vi "Bundler_Selected Element.vi"(7 "Action":T1(ring)=enum."Wire Properties", 11 "Affected Items":T2) -> (0 "Display String":string, 1 "Selected Element Name":string, 2 "index of element":i32, 3 "Selected Element Term Refnum":refnum<vi>, 4 "last element":bool, 6 "first element":bool)   [LabVIEW 2023]
uses:
  top/BundleMagic.ctl
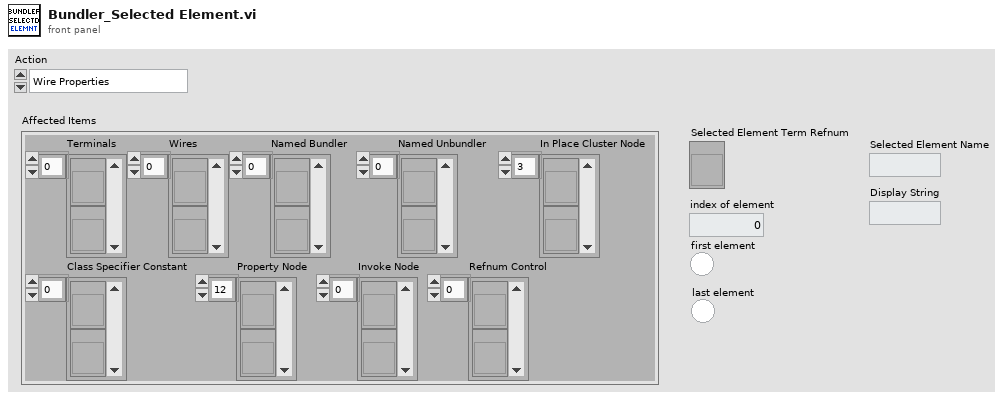
[diagram p1: front panel]
types:
  T1 = enum16{"[NONE]", "Wire Bundle", "Wire Unbundle", "Terminal Unbundle", "Terminal Bundle", "Bundler Move Up", "Bundler Move Down", "Bundler Insert", "Bundler Remove", "Bundler Remove Unwired", "Bundler Rearrange", "In Place Insert", "In Place Remove", "In Place Remove Unwired", "In Place Rearrange", "Wire Properties", "Wire Method", "Terminal Properties", "Terminal Method", "Property Move Up", "Property Move Down", "Properties Insert", "Properties Remove", "Properties Remove Unwired", "Properties Rearrange", "Method Change", "Class for Constant", "Class For Control", "Class For Node", "Class Name to Clipboard"}
  T2 = typedef "BundleMagic.ctl" = cluster{"Terminals":refnum<vi>[], "Wires":refnum<vi>[], "Named Bundler":refnum<vi>[], "Named Unbundler":refnum<vi>[], "In Place Cluster Node":refnum<vi>[], "Class Specifier Constant":refnum<vi>[], "Property Node":refnum<vi>[], "Invoke Node":refnum<vi>[], "Refnum Control":refnum<vi>[]}
  T3 = enum16{"Named Bundler", "Named Unbundler", "In Place", "None"}
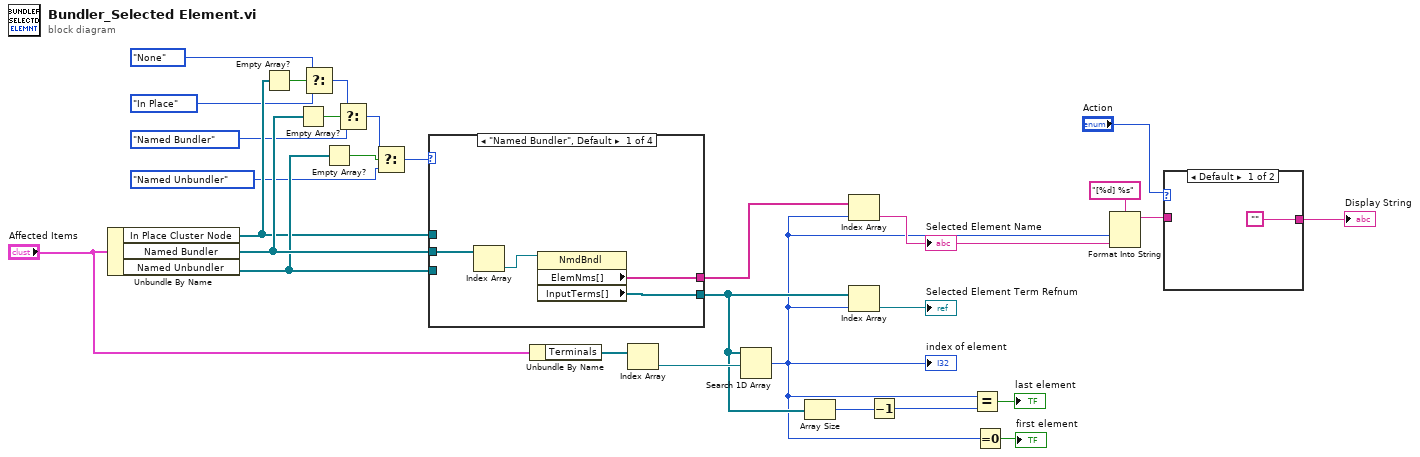
[diagram p0: block diagram]
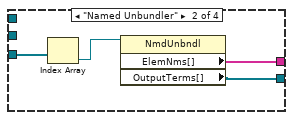
[diagram p3: hidden frame]
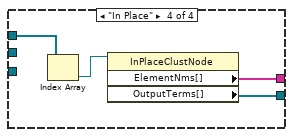
[diagram p5: hidden frame]
diagram:
  n1 = Unbundle By Name("Affected Items") -> ("In Place Cluster Node"=w12:refnum<vi>[], "Named Bundler"=w15:refnum<vi>[], "Named Unbundler"=w14:refnum<vi>[])
  n2 = Empty Array?(array=w12) -> (empty?=w13:bool)
  n3 = Empty Array?(array=w15) -> (empty?=w29:bool)
  n4 = Select(t=T3."None" ("Bundler Type"), s=w13, f=T3."In Place" ("Bundler Type")) -> (s? t:f=w7:T3)
  n5 = Empty Array?(array=w14) -> (empty?=w21:bool)
  n6 = Select(t=w7, s=w29, f=T3."Named Bundler" ("Bundler Type")) -> (s? t:f=w20:T3)
  n7 = Select(t=w20, s=w21, f=T3."Named Unbundler" ("Bundler Type")) -> (s? t:f=w8:T3)
  n8 = case shown="\"Named Bundler\", Default" w8 {
    tunnel: w14 -> [_ w37 _ _]
    tunnel: w15 -> [w33 _ _ _]
    tunnel: [w31 w35 _ w41] -> w24
    tunnel: [w30 w34 _ w40] -> w6
    tunnel: w12 -> [_ _ _ w39]
    frame "Named Bundler", Default {
      n9 = Index Array(array=w33) -> (element=w32:refnum<vi>)  [unwired: 1 in]
      n10 = property class="NmdBndl"(reference=w32) -> ("ElemNms[]"=w31:string[], "InputTerms[]"=w30:refnum<vi>[])  [unwired: 1 in, 2 out]
    }
    frame "Named Unbundler" {
      n11 = Index Array(array=w37) -> (element=w36:refnum<vi>)  [unwired: 1 in]
      n12 = property class="NmdUnbndl"(reference=w36) -> ("ElemNms[]"=w35:string[], "OutputTerms[]"=w34:refnum<vi>[])  [unwired: 1 in, 2 out]
    }
    frame "None" {
    }
    frame "In Place" {
      n13 = Index Array(array=w39) -> (element=w38:refnum<vi>)  [unwired: 1 in]
      n14 = property class="InPlaceClustNode"(reference=w38) -> ("ElementNms[]"=w41:string[], "OutputTerms[]"=w40:refnum<vi>[])  [unwired: 1 in, 2 out]
    }
  }
  n15 = Unbundle By Name("Affected Items") -> ("Terminals"=w27:refnum<vi>[])
  n16 = Index Array(array=w27) -> (element=w26:refnum<vi>)  [unwired: 1 in]
  n17 = Search 1D Array(1D array=w6, element=w26) -> (index of element=w2:i32)  [unwired: 1 in]
  "index of element" <- w2
  n18 = Array Size(array=w6) -> (size(s)=w5:i32)
  n19 = Index Array(array=w24, index=w2) -> (element=w23:string)
  "Selected Element Name" <- w23
  n20 = Index Array(array=w6, index=w2) -> (element=→"Selected Element Term Refnum":refnum<vi>)
  n21 = Decrement(x=w5) -> (x-1=w4:i32)
  n22 = Equal?(x=w2, y=w4) -> (x = y?=→"last element":bool)
  n23 = Equal To 0?(x=w2) -> (x = 0?=→"first element":bool)
  n24 = Format Into String(format string="[%d] %s", w2, w23) -> (resulting string=w17:string)  [unwired: 2 in, 1 out]
  n25 = case shown="Default" "Action" {
    tunnel: ["" w43] -> w18
    tunnel: w17 -> [_ w43]
    frame Default {
    }
    frame "Bundler Insert", "In Place Insert" {
    }
  }
  "Display String" <- w18
